vi "capa espuma.vi"(8 "error in (no error)":errorcluster, 11 "Refnum in":refnum<k21>) -> (0 "error out":errorcluster, 1 "gas holdup":dbl, 2 "Flotation column":dbl, 3 "Refnum out":refnum<k21>, 5 "element":dbl)   [LabVIEW 2013]
uses:
  <vilib>/DAQmx/read.llb/DAQmx Read (Analog 1D DBL NChan 1Samp).vi
panel:
  out "x*y":dbl
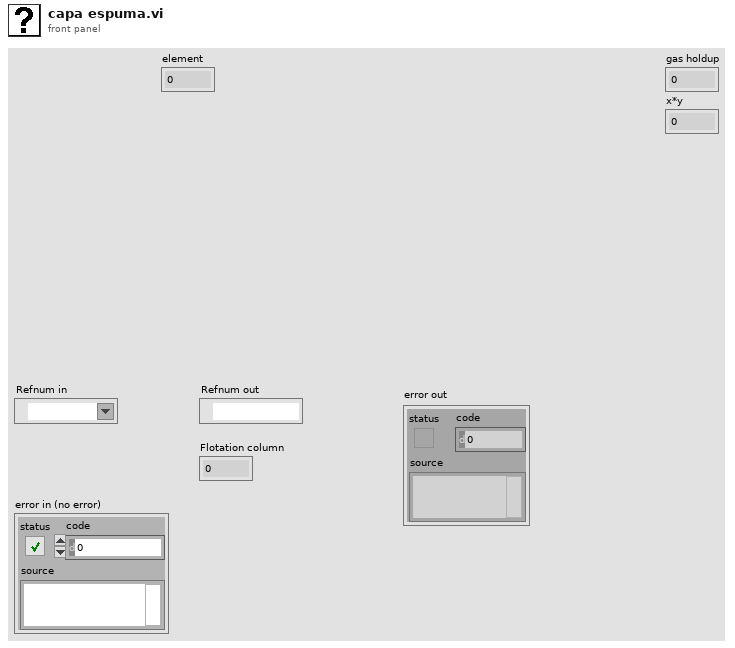
[diagram p1: front panel]
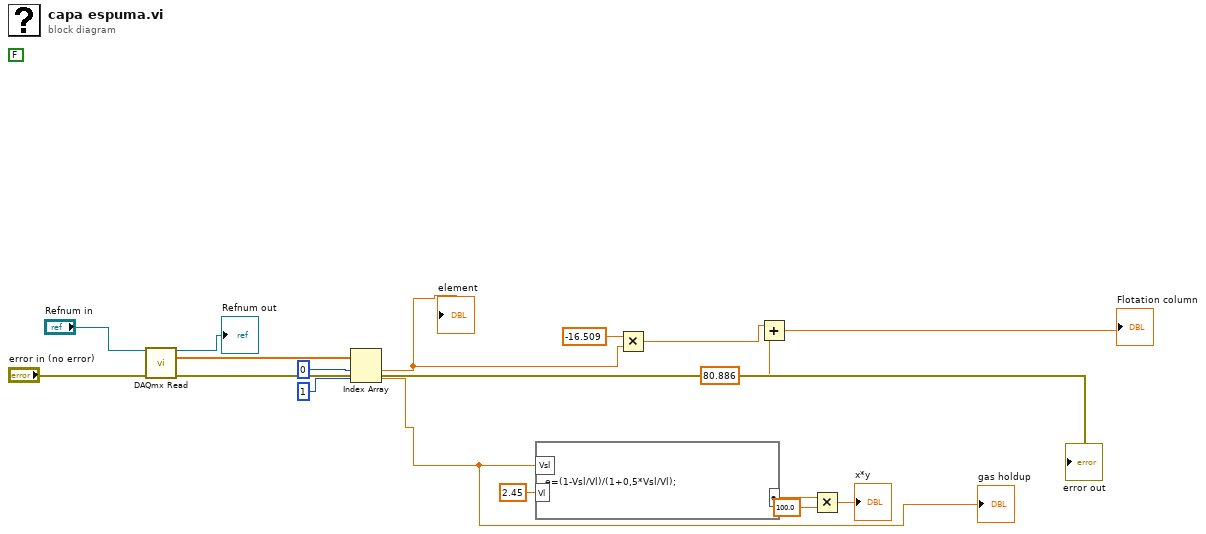
[diagram p0: block diagram]
diagram:
  (unwired) FALSE
  n1 = call-poly <vilib>:"DAQmx Read.vi"("task/channels in"="Refnum in", "error in"="error in (no error)") -> ("task out"=→"Refnum out":refnum<k21>, "data"=w13:dbl[], "error out"=→"error out":errorcluster)  [unwired: 11 in]
  n2 = Index Array(array=w13, index #1=0 ("index"), index #2=1 ("index")) -> (element #1=w1:dbl, element #2=w6:dbl)
  "gas holdup" <- w6
  "element" <- w1
  n3 = formula code="e=(1-Vsl/Vl)/(1+0,5*Vsl/Vl);"("Vsl"=w6, "Vl"=2.45 ("input variable")) -> ("e"=w8:dbl)
  n4 = Multiply(x=-16.509, y=w1) -> (x*y=w4:dbl)
  n5 = Add(x=w4, y=80.886 ("value")) -> (x+y=→"Flotation column":dbl)
  n6 = Multiply(x=w8, y=100.0) -> (x*y=→"x*y":dbl)
